vi "Fiducical Parameters Finder.vi"() -> ()   [LabVIEW 2011]
uses:
  Shared Components/Gantry Class/Gantry Class.lvclass
  Shared Components/gVision API/gVision/gVision.lvlib
panel:
  in  "Fiducial Parameters":T1
  out "error out":errorcluster
  out "ficucial coordinates":cluster{"x":dbl, "y":dbl}[](array[cluster])
  in  "Stop":bool
  out "Result":T2(plugin-control)
  in  "Display Steps":bool
  out "Preview":T2(plugin-control)
  in  "Find Fiducial":bool
  in  "Config Folder":path=path "C:/Users/Husker/Desktop/gantry/Config"
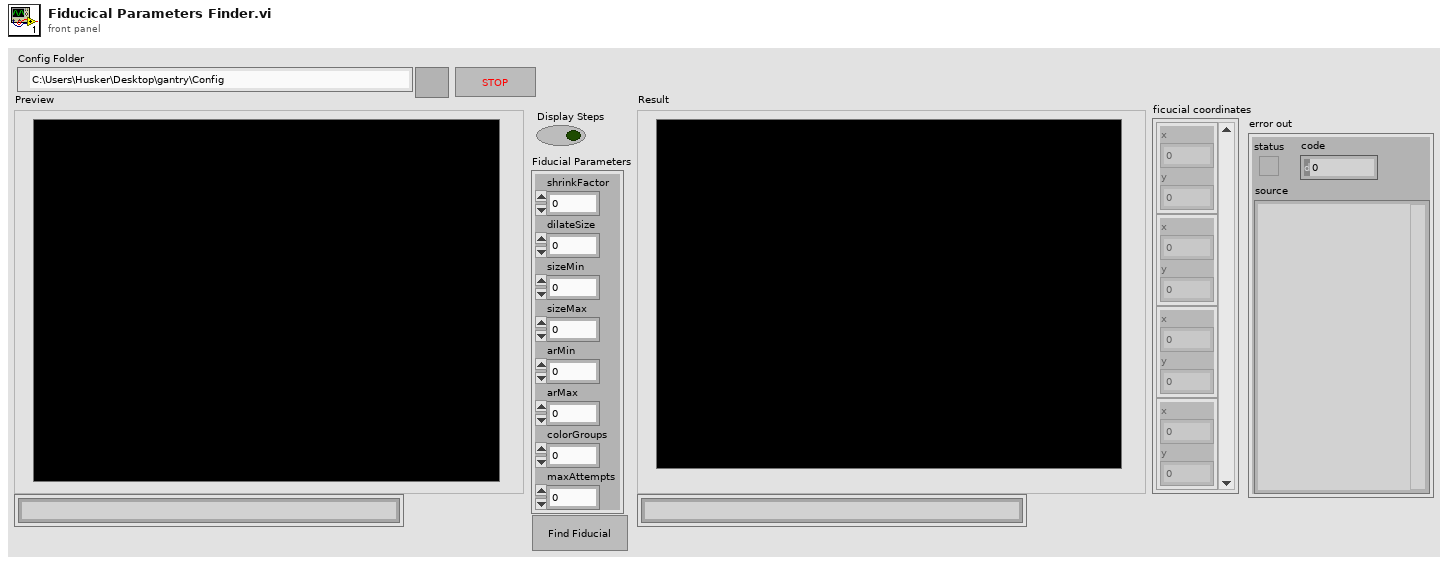
[diagram p1: front panel]
types:
  T1 = cluster{"shrinkFactor":sgl, "dilateSize":i32, "sizeMin":sgl, "sizeMax":sgl, "arMin":sgl, "arMax":sgl, "colorGroups":i32, "maxAttempts":i32}
  T2 = typedef "IMAQ Image.ctl" = refnum<image>
  T3 = cluster{"Left":i32, "Top":i32, "Right":i32, "Bottom":i32}
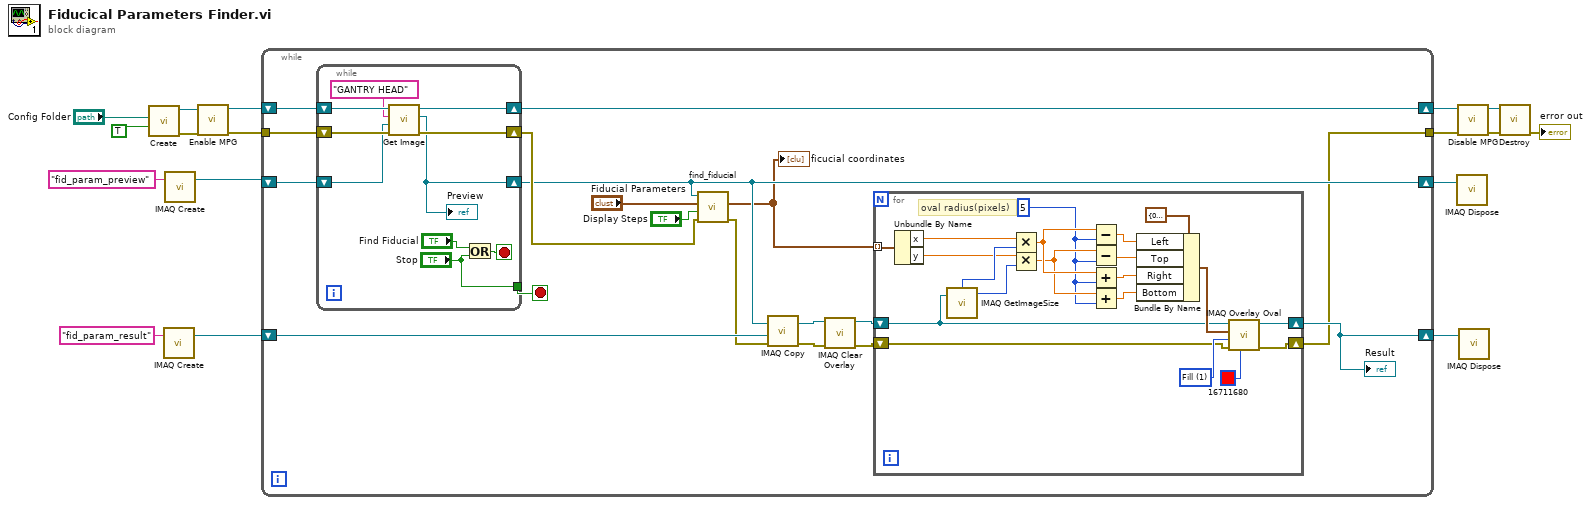
[diagram p0: block diagram]
diagram:
  n1 = call "Create.vi"("HOME?"=TRUE, "Config Folder"="Config Folder") -> ("error out"=w15:errorcluster, "Gantry out"=w14:refnum<class "Gantry Class.lvclass">)  [unwired: 8 in]
  n2 = call "IMAQ Create"("Image Name"="fid_param_result") -> ("New Image"=w7:T2)  [unwired: 4 in, 1 out]
  n3 = call "IMAQ Create"("Image Name"="fid_param_preview") -> ("New Image"=w11:T2)  [unwired: 4 in, 1 out]
  n4 = call-dynamic "Enable MPG.vi"("error in (no error)"=w15, "Gantry Class in"=w14) -> ("error out"=w12:errorcluster, "Gantry Class out"=w13:refnum<class "Gantry Class.lvclass">)  [unwired: 8 in]
  n5 = while {
    tunnel: w12 -> [w35]
    shift-right: [w28] -> w10
    shift-left: w11 -> [w33]
    shift-right: [w30] -> w5
    shift-left: w13 -> [w34]
    shift-right: [w25] -> w6
    shift-left: w7 -> [w27]
    tunnel: [w19] -> w2
    stop <- w29 stop-if-true
    n6 = while {
      shift-right: [w59] -> w28
      shift-left: w33 -> [w62]
      shift-right: [w61] -> w30
      shift-left: w34 -> [w64]
      shift-right: [w60] -> w31
      shift-left: w35 -> [w65]
      tunnel: ["Stop"] -> w29
      stop <- w57 stop-if-true
      n7 = call-dynamic "Get Image.vi"("error in"=w65, "Image In"=w62, "Camera Name"="GANTRY HEAD", "Gantry in"=w64) -> ("error out"=w60:errorcluster, "Image Out"=w59:T2, "Gantry out"=w61:refnum<class "Gantry Class.lvclass">)  [unwired: 4 in, 1 out]
      "Preview" <- w59
      n8 = Or(x="Find Fiducial", y="Stop") -> (x .or. y?=w57:bool)
    }
    n9 = call "find_fiducial.vi"("error in"=w31, "interactive"="Display Steps", "Fiducial Parameters"="Fiducial Parameters", "Image"=w28) -> ("error out"=w24:errorcluster, "coords"=w26:cluster{"x":dbl, "y":dbl}[])  [unwired: 6 in]
    "ficucial coordinates" <- w26
    n10 = call "IMAQ Copy"("error in (no error)"=w24, "Image Dst"=w27, "Image Src"=w28) -> ("error out"=w22:errorcluster, "Image Dst Out"=w23:T2)  [unwired: 3 in]
    n11 = call "IMAQ Clear Overlay"("error in (no error)"=w22, "Image"=w23) -> ("error out"=w20:errorcluster, "Image Out"=w21:T2)  [unwired: 8 in]
    n12 = for {
      tunnel: w26 -> [w51] mode=indexing
      shift-right: [w55] -> w25
      shift-left: w21 -> [w47]
      shift-right: [w49] -> w19
      shift-left: w20 -> [w48]
      w36 = 5
      w50 = u32 1 items=["Frame", "Fill"] ("Drawing Mode (Frame)")
      # "oval radius(pixels)"
      n13 = Unbundle By Name(w51) -> ("x"=w45:dbl, "y"=w43:dbl)
      n14 = call "IMAQ GetImageSize"("Image"=w47) -> ("Y Resolution"=w44:i32, "X Resolution"=w46:i32)  [unwired: 3 in, 1 out]
      n15 = Multiply(x=w45, y=w46) -> (x*y=w38:dbl)
      n16 = Multiply(x=w43, y=w44) -> (x*y=w37:dbl)
      n17 = Subtract(x=w38, y=w36) -> (x-y=w42:dbl)
      n18 = Subtract(x=w37, y=w36) -> (x-y=w41:dbl)
      n19 = Add(x=w38, y=w36) -> (x+y=w40:dbl)
      n20 = Add(x=w37, y=w36) -> (x+y=w39:dbl)
      n21 = Bundle By Name(cluster=T3 {"Left"=0, "Top"=0, "Right"=0, "Bottom"=0} ("Bounding Rectangle"), "Left"=w42, "Top"=w41, "Right"=w40, "Bottom"=w39) -> (w52:T3)
      n22 = call "IMAQ Overlay Oval"("Color"=u32 16711680, "error in (no error)"=w48, "Drawing Mode (Frame)"=w50, "Bounding Rectangle"=w52, "Image"=w47) -> ("error out"=w49:errorcluster, "Image Out"=w55:T2)  [unwired: 5 in]
    }
    "Result" <- w25
  }
  n23 = call "IMAQ Dispose"("Image"=w10) -> ()  [unwired: 5 in, 1 out]
  n24 = call-dynamic "Disable MPG.vi"("error in"=w2, "Gantry in"=w5) -> ("error out"=w4:errorcluster, "Gantry out"=w3:refnum<class "Gantry Class.lvclass">)  [unwired: 8 in]
  n25 = call "IMAQ Dispose"("Image"=w6) -> ()  [unwired: 5 in, 1 out]
  n26 = call "Destroy.vi"("error in"=w4, "Gantry Class in"=w3) -> ("error out"=→"error out":errorcluster)  [unwired: 9 in]
